vi "constructor.vi"(8 "error in (no error)":errorcluster, 10 "device":string) -> (0 "error out":errorcluster, 3 "DDSOutput out":refnum<class "DDSOutput.lvclass">)   [LabVIEW 2011, in "Hardware.lvlib" / "Channels.lvlib" / "DDSOutput.lvclass"]
uses:
  DDSOutput.lvclass
  SpinCore/SpinCore.lvclass
  k3390_AWG/k3390_AWG.lvclass
  CQT_DDS/CQT_DDS.lvclass
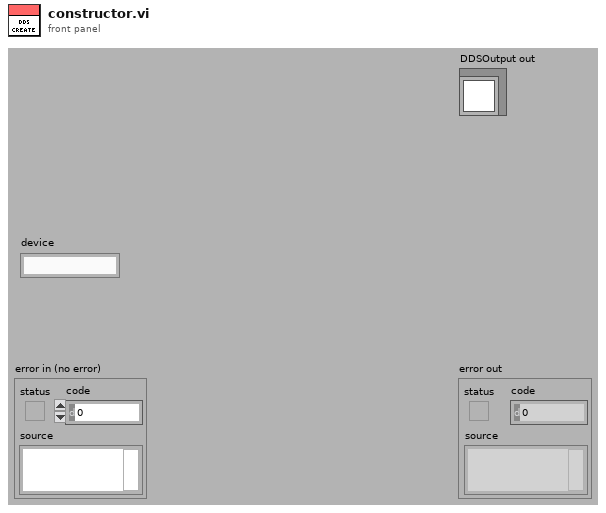
[diagram p1: front panel]
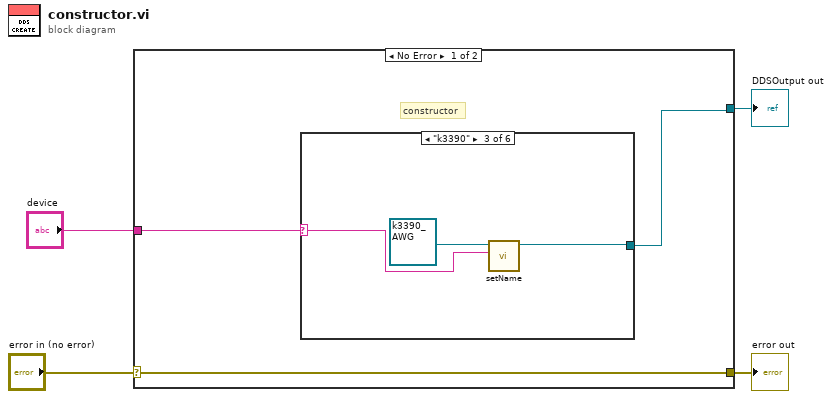
[diagram p0: block diagram]
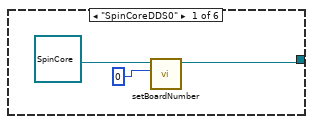
[diagram p2: hidden frame]
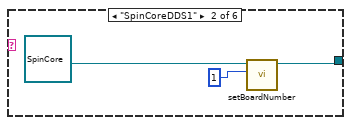
[diagram p3: hidden frame]
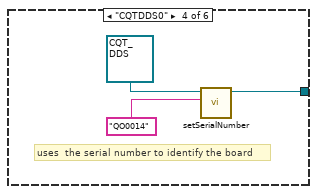
[diagram p4: hidden frame]
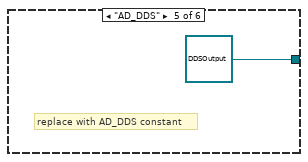
[diagram p5: hidden frame]
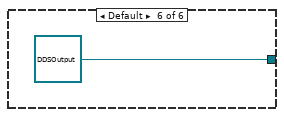
[diagram p6: hidden frame]
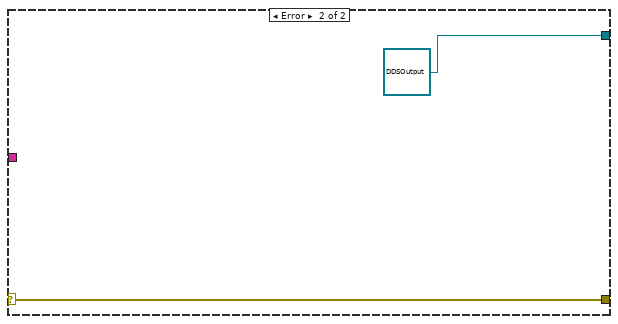
[diagram p7: hidden frame]
diagram:
  n1 = case shown="No Error" "error in (no error)" {
    selector: "error in (no error)" -> [w7 w23]
    tunnel: [w7 w23] -> w3
    tunnel: "device" -> [w6 _]
    tunnel: [w5 refnum<class "DDSOutput.lvclass"> refnum ("DDSOutput in")] -> w1
    frame No Error {
      # "constructor"
      n2 = case shown="\"k3390\"" w6 {
        selector: w6 -> [_ _ w15 _ _ _]
        tunnel: [w9 w12 w14 w17 refnum<class "DDSOutput.lvclass"> refnum ("DDSOutput in") refnum<class "DDSOutput.lvclass"> refnum ("DDSOutput in")] -> w5
        frame "SpinCoreDDS0" {
          n3 = call "setBoardNumber.vi"("boardNumber"=0, "SpinCore in"=refnum<class "SpinCore.lvclass"> refnum ("Hardware:Channels.lvlib:SpinCore.lvclass")) -> ("SpinCore out"=w9:refnum<class "SpinCore.lvclass">)  [unwired: 8 in, 1 out]
        }
        frame "SpinCoreDDS1" {
          n4 = call "setBoardNumber.vi"("boardNumber"=1, "SpinCore in"=refnum<class "SpinCore.lvclass"> refnum ("Hardware:Channels.lvlib:SpinCore.lvclass")) -> ("SpinCore out"=w12:refnum<class "SpinCore.lvclass">)  [unwired: 8 in, 1 out]
        }
        frame "k3390" {
          n5 = call "setName.vi"("name"=w15, "DDSOutput in"=refnum<class "k3390_AWG.lvclass"> refnum ("Hardware:Channels.lvlib:k3390_AWG.lvclass")) -> ("DDSOutput out"=w14:refnum<class "k3390_AWG.lvclass">)  [unwired: 8 in, 1 out]
        }
        frame "CQTDDS0" {
          # "uses  the serial number to identify the board"
          n6 = call "setSerialNumber.vi"("serialNumber"="QO0014", "CQT_DDS in"=refnum<class "CQT_DDS.lvclass"> refnum ("Hardware:Channels.lvlib:CQT_DDS.lvclass")) -> ("CQT_DDS out"=w17:refnum<class "CQT_DDS.lvclass">)  [unwired: 8 in, 1 out]
        }
        frame "AD_DDS" {
          # "replace with AD_DDS constant"
        }
        frame Default {
        }
      }
    }
    frame Error {
    }
  }
  "error out" <- w3
  "DDSOutput out" <- w1
